vi "Close.vi"(8 "error in (no error)":errorcluster caption="entrée d'erreur (pas d'erreur)", 11 "Class UART (Default) en entrée":refnum<class "Class UART (Default).lvclass">) -> (0 "error out":errorcluster caption="sortie d'erreur", 3 "Class UART (Default) en sortie":refnum<class "Class UART (Default).lvclass">)   [LabVIEW 2020, in "Library Instrument & Equipement.lvlib" / "Library UART.lvlib" / "Class UART (Default).lvclass"]
uses:
  Class UART (Default).lvclass
  Class UART (Default).lvclass/Class UART (Default).ctl
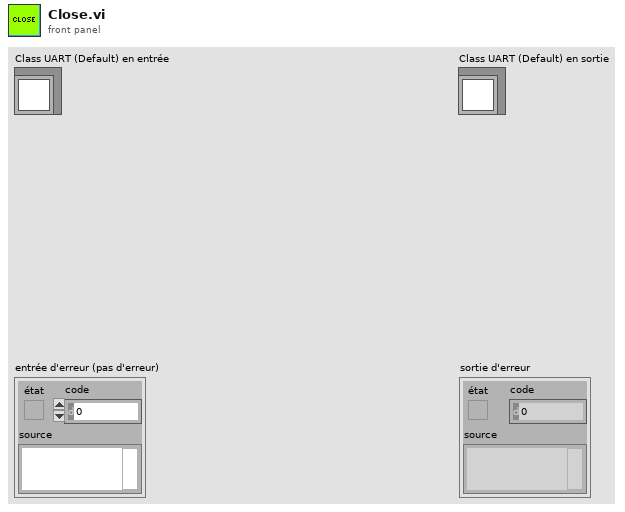
[diagram p1: front panel]
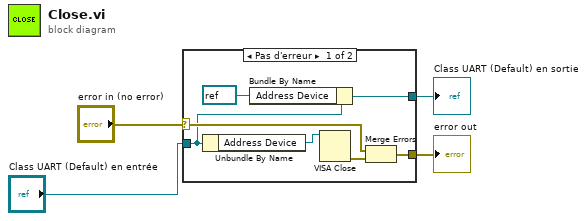
[diagram p0: block diagram]
diagram:
  n1 = case shown="Pas d'erreur" "error in (no error)" {
    selector: "error in (no error)" -> [w11 w13]
    tunnel: [w8 w13] -> w3
    tunnel: [w6 w12] -> w1
    tunnel: "Class UART (Default) en entrée" -> [w10 w12]
    frame No Error {
      n2 = Unbundle By Name(w10) -> ("Address Device"=w9:refnum<visa-resource-name>)
      n3 = Bundle By Name(cluster=w10, "Address Device"=refnum<visa-resource-name> refnum) -> (w6:refnum<class "Class UART (Default).lvclass">)
      n4 = VISA Close(VISA resource name=w9) -> (error out=w7:errorcluster)  [unwired: 1 in]
      n5 = Merge Errors(w11, w7) -> (w8:errorcluster)
    }
    frame Error {
    }
  }
  "error out" <- w3
  "Class UART (Default) en sortie" <- w1
